vi "ABR3-Show Threshold Estimation Work.vi"(7 "work":T1) -> ()   [LabVIEW 2020]
uses:
  ABR3-Threshold Estimation Work.ctl
  ABR3-Threshold Estimation Result.ctl
panel:
  out "Threshold":dbl
  out "Sigmoid":string
  out "Power2":string
  out "graph":cluster{dbl[], dbl[]}[](graph)
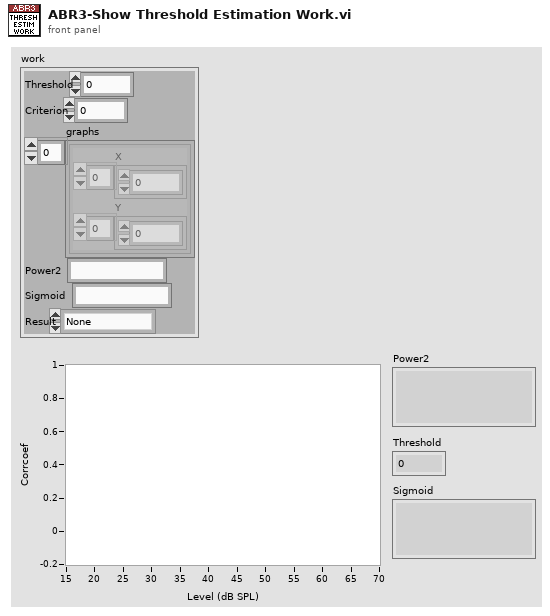
[diagram p1: front panel]
types:
  T1 = typedef "ABR3-Threshold Estimation Work.ctl" = cluster{"Threshold":dbl, "Criterion":dbl, "graphs":cluster{"X":dbl[], "Y":dbl[]}[], "Power2":string, "Sigmoid":string, "Result":T2}
  T2 = typedef "ABR3-Threshold Estimation Result.ctl" = enum16{"None", "Power", "Sigmoid", "Power (noisy)", "Suprathreshold", "Invalid"}
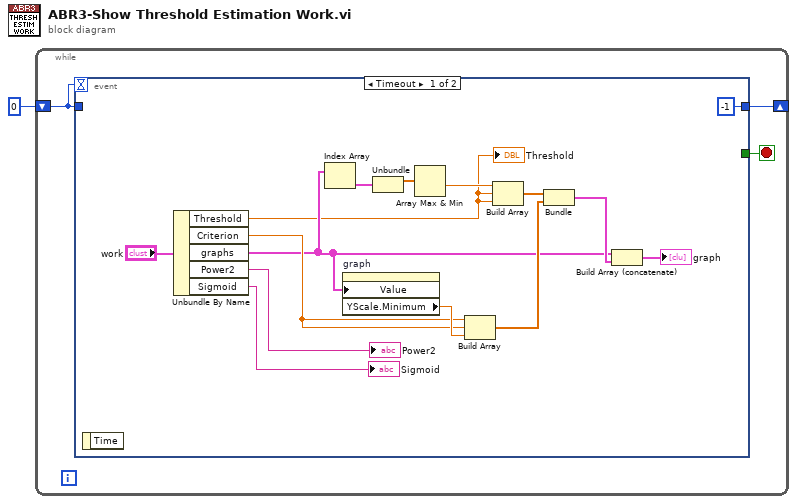
[diagram p0: block diagram]
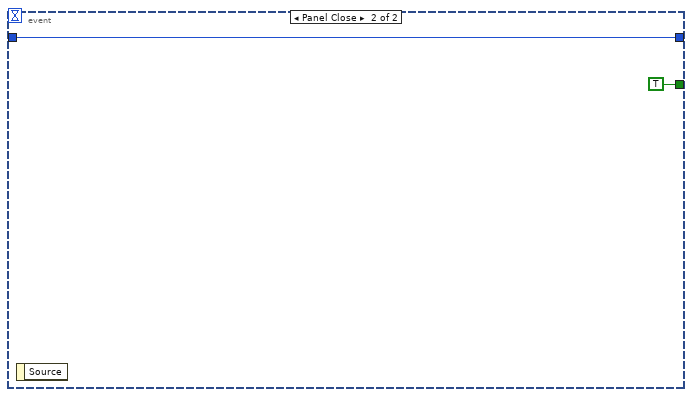
[diagram p2: hidden frame]
diagram:
  n1 = while {
    shift-right: [w3] -> _
    shift-left: 0 -> [w4]
    stop <- w2 stop-if-true
    n2 = event shown="[0] Timeout" {
      selector: _ -> [_ _]
      dyn-events: _ -> [_ _]
      timeout: w4 -> [_ _]
      tunnel: w4 -> [_ w21]
      tunnel: [-1 w21] -> w3
      tunnel: [_ TRUE] -> w2
      event Timeout {
        n3 = event-data() -> ()  [unwired: 1 in, 1 out]
        n4 = Unbundle By Name("work") -> ("Threshold"=w5:dbl, "Criterion"=w10:dbl, "graphs"=w7:cluster{"X":dbl[], "Y":dbl[]}[], "Power2"=→"Power2":string, "Sigmoid"=→"Sigmoid":string)
        "Threshold" <- w5
        n5 = Index Array(array=w7) -> (element=w12:cluster{"X":dbl[], "Y":dbl[]})  [unwired: 1 in]
        n6 = property on="graph" class="XYGraph (strict)"("Value"=w7) -> ("YScale.Minimum"=w19:dbl)  [unwired: 2 in, 2 out]
        n7 = Unbundle(w12) -> ("X"=w11:dbl[])  [unwired: 1 out]
        n8 = Array Max & Min(array=w11) -> (min value=w18:dbl)  [unwired: 3 out]
        n9 = Build Array(w10, w10, w19) -> (w16:dbl[])
        n10 = Build Array(w18, w5, w5) -> (w17:dbl[])
        n11 = Bundle(w17, w16) -> (w15:cluster{dbl[], dbl[]})  [unwired: 1 in]
        n12 = Build Array (concatenate)(w7, w15) -> (→"graph":cluster{"X":dbl[], "Y":dbl[]}[])
      }
      event Panel Close {
        n13 = event-data() -> ()  [unwired: 1 in, 1 out]
      }
    }
  }
